vi "updateMission.vi"(8 "error in (no error)":errorcluster, 11 "MissionQueue in":refnum<class "MissionQueue.lvclass">) -> (0 "error out":errorcluster, 2 "CurrentMission":refnum<class "GenericMission.lvclass">, 3 "MissionQueue out":refnum<class "MissionQueue.lvclass">)   [LabVIEW 2011, in "MissionQueue.lvclass"]
uses:
  MissionQueue.lvclass
  Missions/GenericMission/GenericMission.lvclass
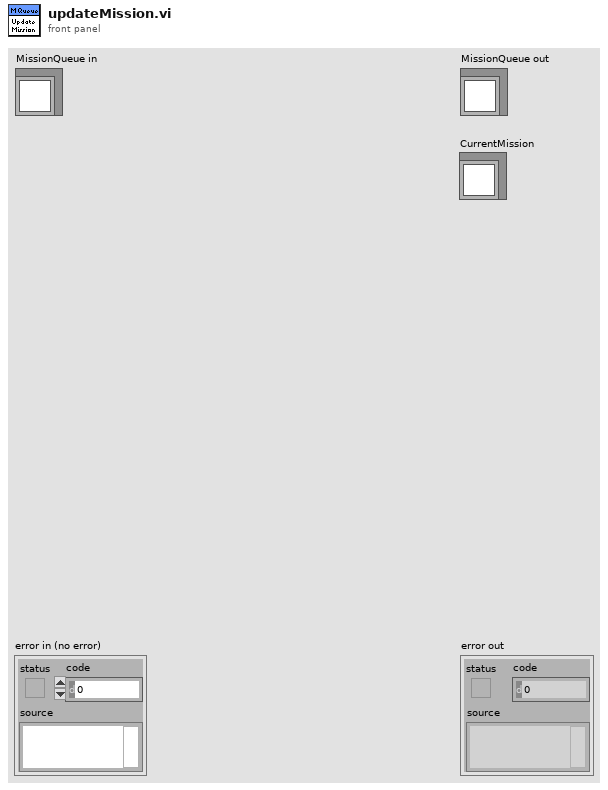
[diagram p1: front panel]
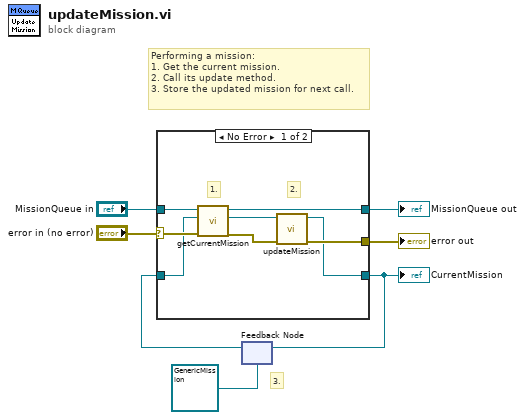
[diagram p0: block diagram]
diagram:
  # "3."
  # "Performing a mission:\n1. Get the current mission.\n2. Call its update method.\n3. Store the updated mission for next call."
  n1 = feedback #1(refnum<class "GenericMission.lvclass"> refnum ("GenericMission out")) -> (w1:refnum<class "GenericMission.lvclass">)
  n2 = case shown="No Error" "error in (no error)" {
    selector: "error in (no error)" -> [w14 w18]
    tunnel: [w10 w18] -> w6
    tunnel: [w11 w17] -> w4
    tunnel: "MissionQueue in" -> [w15 w17]
    tunnel: [w9 w16] -> w2
    tunnel: w1 -> [w8 w16]
    frame No Error {
      # "2."
      # "1."
      n3 = call "getCurrentMission.vi"("error in (no error)"=w14, "Current Mission In"=w8, "MissionQueue in"=w15) -> ("error out"=w12:errorcluster, "Mission Out"=w13:refnum<class "GenericMission.lvclass">, "MissionQueue out"=w11:refnum<class "MissionQueue.lvclass">)  [unwired: 6 in]
      n4 = call-dynamic "updateMission.vi"("error in (no error)"=w12, "GenericMission in"=w13) -> ("error out"=w10:errorcluster, "GenericMission out"=w9:refnum<class "GenericMission.lvclass">)  [unwired: 8 in]
    }
    frame Error {
    }
  }
  "error out" <- w6
  "MissionQueue out" <- w4
  "CurrentMission" <- w2
  n5 = feedback-in #1(w2) -> ()
